vi "Calculate Slope and Intercept.vi"(8 "y2":dbl, 9 "x2":dbl, 10 "y1":dbl, 11 "x1":dbl) -> (1 "y-intercept":dbl, 2 "slope":dbl)   [LabVIEW 2018]
doc: "Inputs are x,y for 2 distinct points. Outputs are linear slope and y-intercept for the line joining the 2 points."
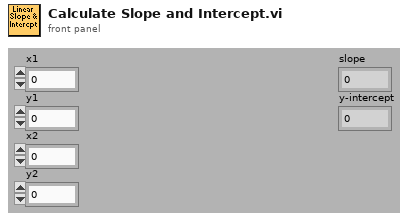
[diagram p1: front panel]
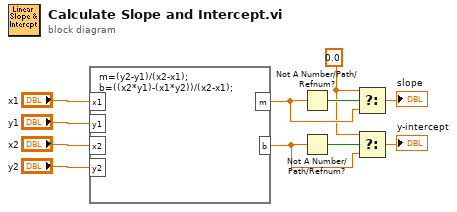
[diagram p0: block diagram]
diagram:
  w3 = 0.0 ("t")
  n1 = formula code="m=(y2-y1)/(x2-x1);\nb=((x2*y1)-(x1*y2))/(x2-x1);"("x1"="x1", "y1"="y1", "x2"="x2", "y2"="y2") -> ("m"=w5:dbl, "b"=w4:dbl)
  n2 = Not A Number/Path/Refnum?(number/path/refnum=w5) -> (NaN/Path/Refnum?=w6:bool)
  n3 = Not A Number/Path/Refnum?(number/path/refnum=w4) -> (NaN/Path/Refnum?=w7:bool)
  n4 = Select(t=w3, s=w6, f=w5) -> (s? t:f=→"slope":dbl)
  n5 = Select(t=w3, s=w7, f=w4) -> (s? t:f=→"y-intercept":dbl)
